vi "Create New Panel.vi"(8 "error in (no error)":errorcluster, 11 "Item_Refnums_Array In":T1[](array[typedef])) -> (0 "error out":errorcluster, 3 "Item_Refnums_Array Out":T1[](array[typedef]))   [LabVIEW 2013, in "UI Panels.lvlib" / "Panels_XControl.xctl"]
uses:
  Panels_XControl.xctl
  Controls/References/Panel_Refnums.ctl
  Controls/Panel_Command_Enum.ctl
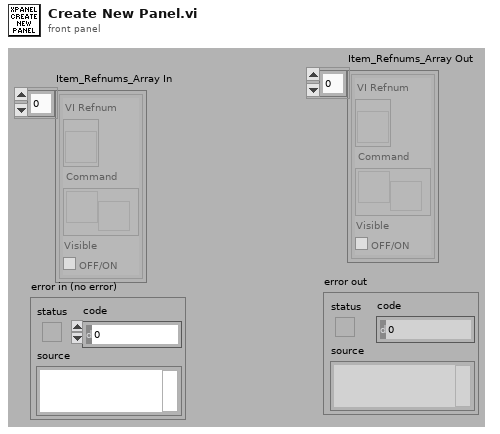
[diagram p1: front panel]
types:
  T1 = typedef "UI Panels.lvlib/Panels_XControl.xctl/Panel_Refnums.ctl" = cluster{"VI Refnum":refnum<vi>, "Command":refnum<user-event>, "Visible":bool}
  T2 = typedef "UI Panels.lvlib/Panels_XControl.xctl/Panel_Command_Enum.ctl" = enum16{"Idle", "Remove & Stop", "Add Item", "Delete Item", "Delete All", "Insert into Subpanel", "Register Menu Events", "Update Value", "Remove from Subpanel", "Set Title", "Set Menu Items", "Insert SubPanel", "Set Splitter Position", "Set Splitter Properties", "Add Menu Items"}
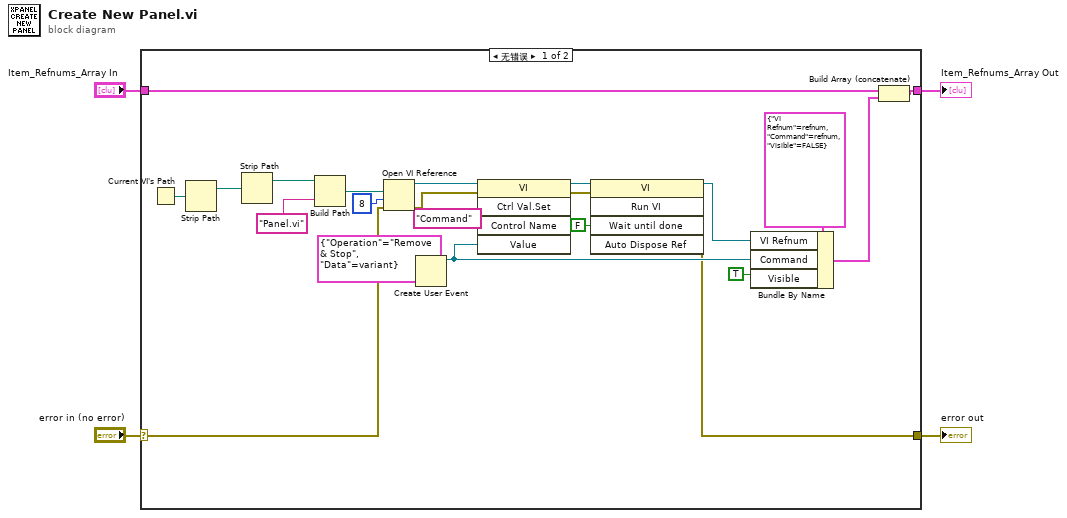
[diagram p0: block diagram]
diagram:
  n1 = case shown="无错误" "error in (no error)" {
    selector: "error in (no error)" -> [w14 w28]
    tunnel: [w26 w27] -> w4
    tunnel: "Item_Refnums_Array In" -> [w13 w27]
    tunnel: [w9 w28] -> w1
    frame No Error {
      w23 = FALSE ("Wait Until Done")
      n2 = Current VI's Path() -> (path=w20:path)
      n3 = Strip Path(path=w20) -> (stripped path=w12:path)  [unwired: 1 out]
      n4 = Strip Path(path=w12) -> (stripped path=w19:path)  [unwired: 1 out]
      n5 = Build Path(base path=w19, name or relative path="Panel.vi") -> (appended path=w17:path)
      n6 = Open VI Reference(vi path=w17, options=8, error in (no error)=w14) -> (vi reference=w8:refnum<vi>, error out=w6:errorcluster)  [unwired: 3 out]
      n7 = Create User Event(user event datatype=cluster{"Operation":T2, "Data":variant} {"Operation"=enum."Remove & Stop", "Data"=variant} ("Item_Command")) -> (user event=w10:refnum<user-event>)  [unwired: 1 in, 1 out]
      n8 = invoke class="VI" method="Ctrl Val.Set"(reference=w8, error in=w6, "Control Name"="Command", "Value"=w10) -> (reference out=w7:refnum<vi>, error out=w5:errorcluster)  [unwired: 1 in, 3 out]
      n9 = invoke class="VI" method="Run VI"(reference=w7, error in=w5, "Wait until done"=w23, "Auto Dispose Ref"=w23) -> (reference out=w15:refnum<vi>, error out=w9:errorcluster)  [unwired: 1 in, 3 out]
      n10 = Bundle By Name(cluster=T1 {"VI Refnum"=refnum, "Command"=refnum, "Visible"=FALSE} ("Item_Refnums"), "VI Refnum"=w15, "Command"=w10, "Visible"=TRUE) -> (w22:T1)
      n11 = Build Array (concatenate)(w13, w22) -> (w26:T1[])
    }
    frame Error {
    }
  }
  "Item_Refnums_Array Out" <- w4
  "error out" <- w1
